vi "ObtainQueue.vi"(6 "ModuleID":i32, 8 "error in (no error)":errorcluster, 10 "ModuleName":string) -> (0 "error out":errorcluster, 3 "MessageQueue":refnum<queue>)   [LabVIEW 2014, in "DigitizerModule.lvlib"]
uses:
  DigitizerModule.lvlib
  PublicAPI/Arguments/Messages/clMessage.ctl
panel:
  # "This obtaind a queue and\nenqueues the \"Initialize\"\nMessage"
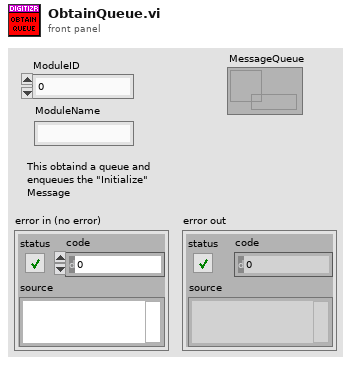
[diagram p1: front panel]
types:
  T1 = typedef "DigitizerModule.lvlib/clMessage.ctl" = cluster{"Message":string, "Message Data":variant}
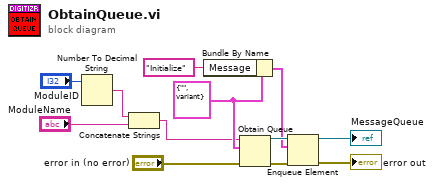
[diagram p0: block diagram]
diagram:
  w10 = T1 {"Message"="", "Message Data"=variant} ("clMessage")
  n1 = Number To Decimal String(number="ModuleID") -> (decimal integer string=w2:string)  [unwired: 1 in]
  n2 = Concatenate Strings(w2, "ModuleName") -> (w1:string)
  n3 = Bundle By Name(cluster=w10, "Message"="Initialize") -> (w8:T1)
  n4 = Obtain Queue(name (unnamed)=w1, element data type=w10, error in (no error)="error in (no error)") -> (queue out=w11:refnum<queue>, error out=w7:errorcluster)  [unwired: 2 in, 1 out]
  n5 = Enqueue Element(queue=w11, element=w8, error in (no error)=w7) -> (queue out=→"MessageQueue":refnum<queue>, error out=→"error out":errorcluster)  [unwired: 1 in, 1 out]
